vi "Build_Asylum_CaptureImage.vi"(8 "error in (no error)":errorcluster, 11 "waveName":string) -> (0 "error out":errorcluster, 3 "Command":string)   [LabVIEW 2019]
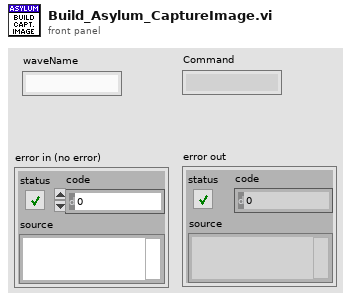
[diagram p1: front panel]
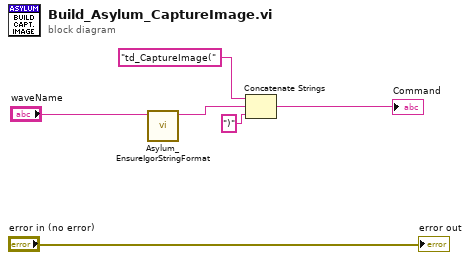
[diagram p0: block diagram]
diagram:
  n1 = call "Asylum_EnsureIgorStringFormat.vi"("Value"="waveName") -> ("Value"=w3:string)  [unwired: 9 in, 1 out]
  n2 = Concatenate Strings("td_CaptureImage(" ("string"), w3, ")" ("string")) -> (→"Command":string)
  "error out" <- "error in (no error)"
